vi "array -- smart enum.vi"(6 "Array of keys":string[](array[string]), 7 "hash action":T1, 9 "index IN":i32, 10 "hash key":string, 11 "hash":refnum<vi>) -> (0 "found?":bool, 1 "index OUT":i32, 2 "hash key OUT":string, 3 "hash OUT":refnum<vi>, 4 "Array of keys OUT":string[](array[string]))   [LabVIEW 2012]
uses:
  hash action control.ctl
  stack action -- control.ctl
panel:
  in  "angle":u16(ring) items=["-54", "-49.5", "-45", "-40.5", "-36", "-27", "-18", "-9", "0", "9", "18", "27", "36", "40.5", "45", "49.5", "54", "58.5", "63"]
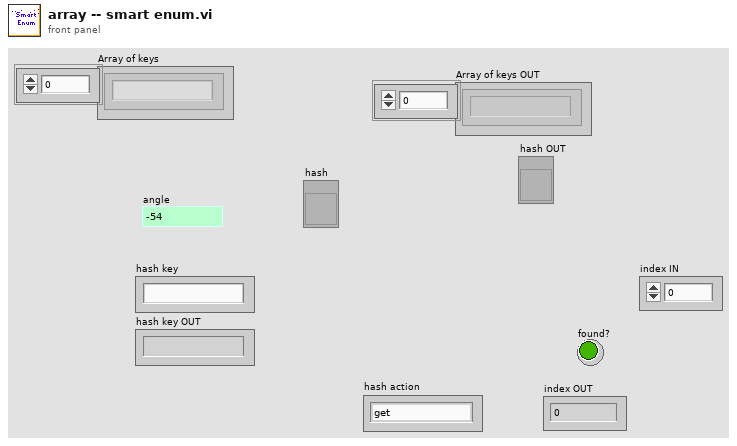
[diagram p1: front panel]
types:
  T1 = typedef "hash action control.ctl" = enum16{"get", "new", "--void", "delete", "delete all", "set", "--delete if exists", "--create if not there", "list keys", "index forw", "index back", "check", "index set", "find key"}
  T2 = typedef "stack action -- control.ctl" = enum16{"push", "pop", "check", "init"}
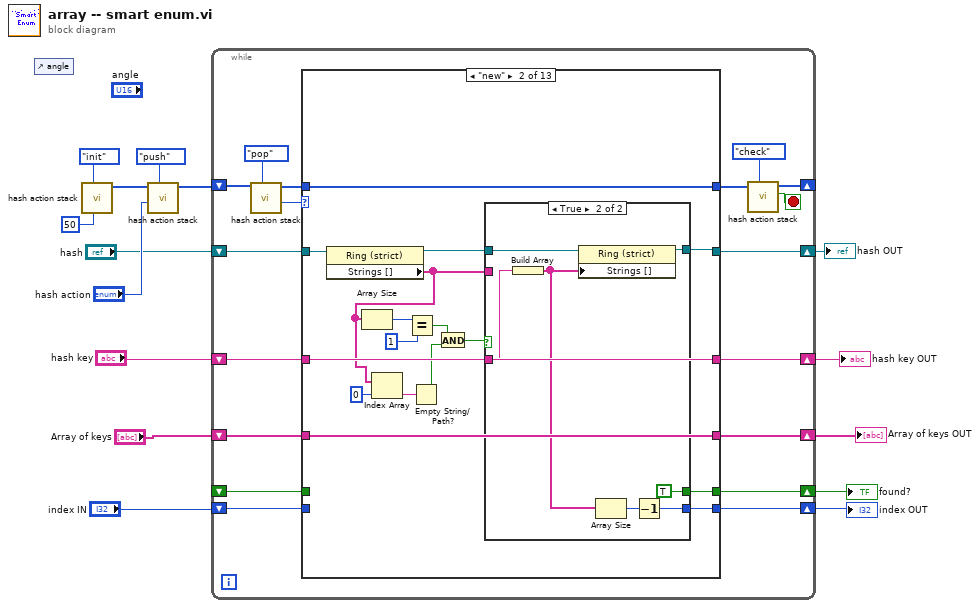
[diagram p0: block diagram]
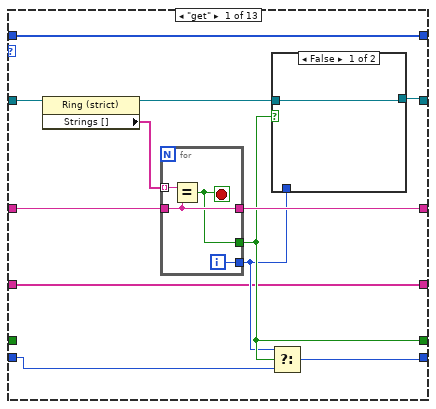
[diagram p2: hidden frame]
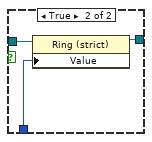
[diagram p3: hidden frame]
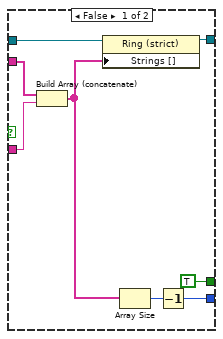
[diagram p4: hidden frame]
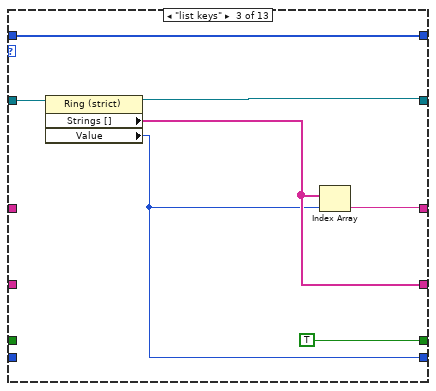
[diagram p5: hidden frame]
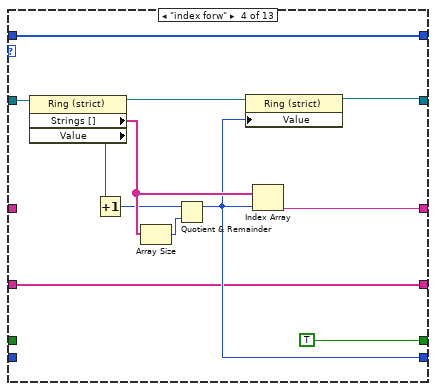
[diagram p6: hidden frame]
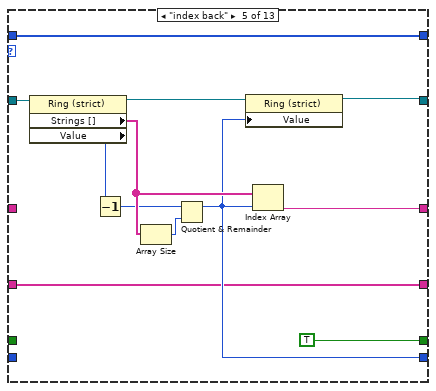
[diagram p7: hidden frame]
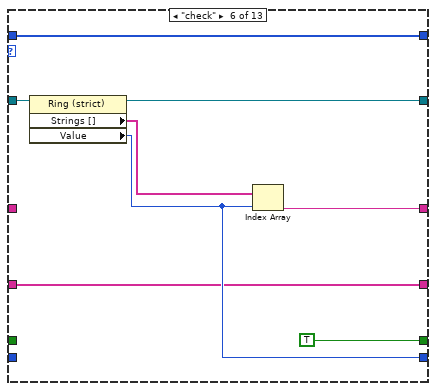
[diagram p8: hidden frame]
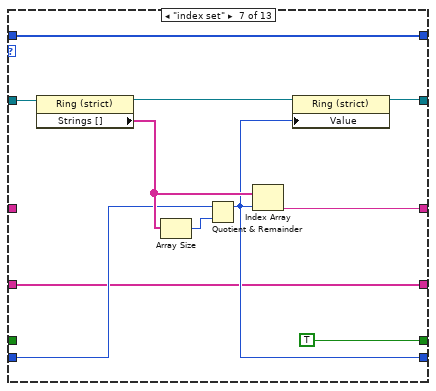
[diagram p9: hidden frame]
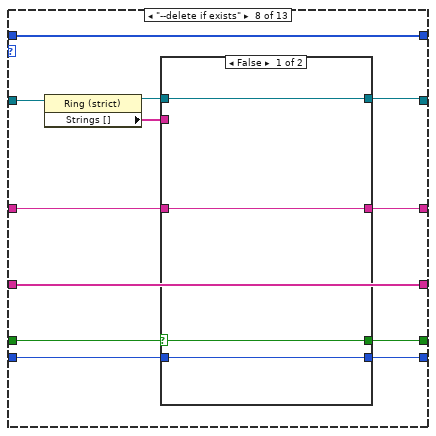
[diagram p10: hidden frame]
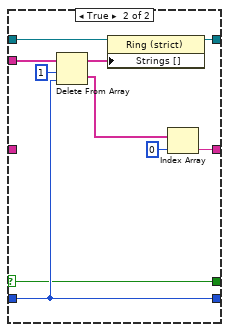
[diagram p11: hidden frame]
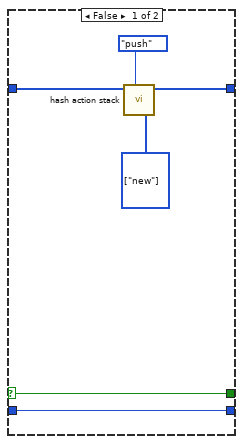
[diagram p13: hidden frame]
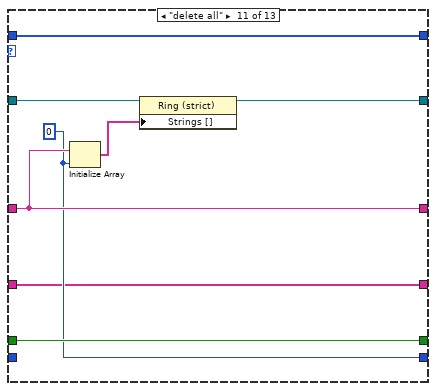
[diagram p15: hidden frame]
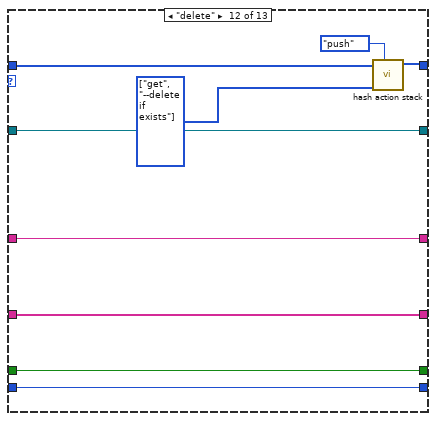
[diagram p16: hidden frame]
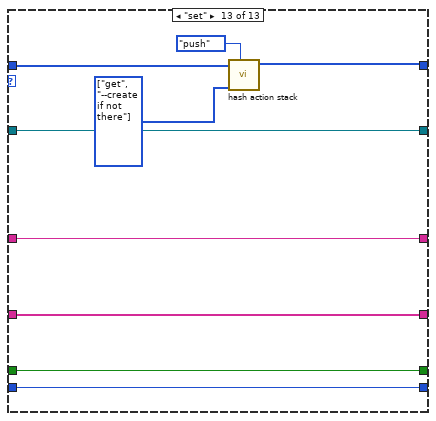
[diagram p17: hidden frame]
diagram:
  n1 = control-ref of="angle"() -> ()  [unwired: 1 out]
  n2 = call "hash action stack.vi"("init size"=50 ("dimension size"), "stack action"=stack_action_--_control."init") -> ("command stack out"=w11:T1[])  [unwired: 7 in, 2 out]
  n3 = call "hash action stack.vi"("stack action"=stack_action_--_control."push", "hash action"="hash action", "command stack"=w11) -> ("command stack out"=w13:T1[])  [unwired: 6 in, 2 out]
  n4 = while {
    shift-right: [w27] -> _
    shift-left: w13 -> [w26]
    shift-right: [w24] -> w8
    shift-left: "index IN" -> [w19]
    shift-right: [w25] -> w9
    shift-left: _ -> [w20]
    shift-right: [w18] -> w3
    shift-left: "hash" -> [w21]
    shift-right: [w23] -> w6
    shift-left: "hash key" -> [w22]
    shift-right: [w17] -> w2
    shift-left: "Array of keys" -> [w16]
    stop <- w28 stop-if-true
    n5 = call "hash action stack.vi"("stack action"=stack_action_--_control."pop", "command stack"=w26) -> ("cursor window action out"=w29:T1, "command stack out"=w32:T1[])  [unwired: 7 in, 1 out]
    n6 = case shown="\"new\"" w29 {
      tunnel: w32 -> [w45 w69 w91 w103 w115 w123 w134 w146 w164 w184 w192 w196 w205]
      tunnel: [w45 w69 w91 w103 w115 w123 w134 w146 w163 w184 w192 w195 w204] -> w30
      tunnel: w21 -> [w42 w67 w89 w101 w113 w121 w132 w139 w162 w180 w190 w194 w203]
      tunnel: w22 -> [w44 w64 _ _ _ _ _ w140 w169 w183 w189 w201 w210]
      tunnel: [w38 w68 TRUE TRUE TRUE TRUE TRUE w142 w165 w182 w191 w200 w209] -> w25
      tunnel: [w40 w63 w86 w93 w105 w118 w125 w143 w166 w181 w186 w199 w208] -> w24
      tunnel: [w43 w64 w85 w97 w109 w120 w131 w141 w169 w183 w189 w201 w210] -> w23
      tunnel: w20 -> [_ _ _ _ _ _ _ w144 w167 w182 w191 w200 w209]
      tunnel: w19 -> [w39 _ _ _ _ _ w128 w145 w168 w181 _ w199 w208]
      tunnel: [w36 w65 w88 w99 w111 w117 w126 w136 w162 w180 w187 w194 w203] -> w18
      tunnel: [w34 w62 w87 w92 w104 w116 w124 w135 w161 w179 w185 w193 w202] -> w17
      tunnel: w16 -> [w34 w62 _ w92 w104 w116 w124 w135 w161 w179 w185 w193 w202]
      frame "get" {
        n7 = property class="Ring (strict)"(reference=w42) -> (reference out=w37:refnum<vi>, "Strings []"=w41:string[])  [unwired: 1 in, 1 out]
        n8 = for {
          tunnel: w44 -> [w52]
          tunnel: [w52] -> w43
          tunnel: w41 -> [w50] mode=indexing
          tunnel: [w53] -> w35
          tunnel: [w51] -> w38
          i -> [w53]
          stop <- w51 stop-if-true
          n9 = Equal?(x=w50, y=w52) -> (x = y?=w51:bool)
        }
        n10 = case shown="False" w38 {
          tunnel: w37 -> [w46 w49]
          tunnel: [w46 w48] -> w36
          tunnel: w35 -> [_ w47]
          frame False {
          }
          frame True {
            n11 = property class="Ring (strict)"(reference=w49, "Value"=w47) -> (reference out=w48:refnum<vi>)  [unwired: 1 in, 1 out]
          }
        }
        n12 = Select(t=w35, s=w38, f=w39) -> (s? t:f=w40:i32)
      }
      frame "new" {
        n13 = property class="Ring (strict)"(reference=w67) -> (reference out=w66:refnum<vi>, "Strings []"=w59:string[])  [unwired: 1 in, 1 out]
        n14 = Array Size(array=w59) -> (size(s)=w61:i32)
        n15 = Index Array(array=w59, index=0) -> (element=w57:string)
        n16 = Equal?(x=w61, y=1) -> (x = y?=w56:bool)
        n17 = Empty String/Path?(string/path=w57) -> (empty?=w55:bool)
        n18 = And(x=w56, y=w55) -> (x .and. y?=w54:bool)
        n19 = case shown="True" w54 {
          tunnel: [TRUE TRUE] -> w68
          tunnel: w66 -> [w75 w82]
          tunnel: [w74 w81] -> w65
          tunnel: w64 -> [w73 w80]
          tunnel: w59 -> [w72 _]
          tunnel: [w71 w79] -> w63
          frame False {
            n20 = Build Array (concatenate)(w72, w73) -> (w70:string[])
            n21 = property class="Ring (strict)"(reference=w75, "Strings []"=w70) -> (reference out=w74:refnum<vi>)  [unwired: 1 in, 1 out]
            n22 = Array Size(array=w70) -> (size(s)=w77:i32)
            n23 = Decrement(x=w77) -> (x-1=w71:i32)
          }
          frame True {
            n24 = Build Array(w80) -> (w78:string[])
            n25 = property class="Ring (strict)"(reference=w82, "Strings []"=w78) -> (reference out=w81:refnum<vi>)  [unwired: 1 in, 1 out]
            n26 = Array Size(array=w78) -> (size(s)=w84:i32)
            n27 = Decrement(x=w84) -> (x-1=w79:i32)
          }
        }
      }
      frame "list keys" {
        n28 = property class="Ring (strict)"(reference=w89) -> (reference out=w88:refnum<vi>, "Strings []"=w87:string[], "Value"=w86:u16)  [unwired: 1 in, 1 out]
        n29 = Index Array(array=w87, index=w86) -> (element=w85:string)
      }
      frame "index forw" {
        n30 = property class="Ring (strict)"(reference=w101) -> (reference out=w100:refnum<vi>, "Strings []"=w96:string[], "Value"=w98:u16)  [unwired: 1 in, 1 out]
        n31 = Increment(x=w98) -> (x+1=w95:u16)
        n32 = Array Size(array=w96) -> (size(s)=w94:i32)
        n33 = Quotient & Remainder(x=w95, y=w94) -> (x-y*floor(x/y)=w93:i32)  [unwired: 1 out]
        n34 = property class="Ring (strict)"(reference=w100, "Value"=w93) -> (reference out=w99:refnum<vi>)  [unwired: 1 in, 1 out]
        n35 = Index Array(array=w96, index=w93) -> (element=w97:string)
      }
      frame "index back" {
        n36 = property class="Ring (strict)"(reference=w113) -> (reference out=w112:refnum<vi>, "Strings []"=w108:string[], "Value"=w110:u16)  [unwired: 1 in, 1 out]
        n37 = Decrement(x=w110) -> (x-1=w107:u16)
        n38 = Array Size(array=w108) -> (size(s)=w106:i32)
        n39 = Quotient & Remainder(x=w107, y=w106) -> (x-y*floor(x/y)=w105:i32)  [unwired: 1 out]
        n40 = property class="Ring (strict)"(reference=w112, "Value"=w105) -> (reference out=w111:refnum<vi>)  [unwired: 1 in, 1 out]
        n41 = Index Array(array=w108, index=w105) -> (element=w109:string)
      }
      frame "check" {
        n42 = property class="Ring (strict)"(reference=w121) -> (reference out=w117:refnum<vi>, "Strings []"=w119:string[], "Value"=w118:u16)  [unwired: 1 in, 1 out]
        n43 = Index Array(array=w119, index=w118) -> (element=w120:string)
      }
      frame "index set" {
        n44 = property class="Ring (strict)"(reference=w132) -> (reference out=w127:refnum<vi>, "Strings []"=w130:string[])  [unwired: 1 in, 1 out]
        n45 = Array Size(array=w130) -> (size(s)=w129:i32)
        n46 = Quotient & Remainder(x=w128, y=w129) -> (x-y*floor(x/y)=w125:i32)  [unwired: 1 out]
        n47 = Index Array(array=w130, index=w125) -> (element=w131:string)
        n48 = property class="Ring (strict)"(reference=w127, "Value"=w125) -> (reference out=w126:refnum<vi>)  [unwired: 1 in, 1 out]
      }
      frame "--delete if exists" {
        n49 = property class="Ring (strict)"(reference=w139) -> (reference out=w137:refnum<vi>, "Strings []"=w138:string[])  [unwired: 1 in, 1 out]
        n50 = case shown="False" w144 {
          selector: w144 -> [w150 w158]
          tunnel: w145 -> [w149 w159]
          tunnel: [w149 w159] -> w143
          tunnel: [w150 w158] -> w142
          tunnel: [w148 w151] -> w141
          tunnel: w140 -> [w148 _]
          tunnel: w138 -> [_ w156]
          tunnel: w137 -> [w147 w155]
          tunnel: [w147 w154] -> w136
          frame False {
          }
          frame True {
            n51 = Delete From Array(array=w156, length=1, index=w159) -> (deleted portion=w152:string[], array with subset deleted=w153:string[])
            n52 = property class="Ring (strict)"(reference=w155, "Strings []"=w153) -> (reference out=w154:refnum<vi>)  [unwired: 1 in, 1 out]
            n53 = Index Array(array=w152, index=0) -> (element=w151:string)
          }
        }
      }
      frame "--create if not there" {
        n54 = case shown="True" w167 {
          selector: w167 -> [w174 w178]
          tunnel: w168 -> [w175 w176]
          tunnel: [w175 w176] -> w166
          tunnel: [w174 w178] -> w165
          tunnel: w164 -> [w172 w177]
          tunnel: [w171 w177] -> w163
          frame False {
            w170 = T1[] [enum."new"] items=["get", "new", "--void", "delete", "delete all", "set", "--delete if exists", "--create if not there", "list keys", "index forw", "index back", "check", "index set", "find key"] ("hash action list")
            n55 = call "hash action stack.vi"("stack action"=stack_action_--_control."push", "hash action list"=w170, "command stack"=w172) -> ("command stack out"=w171:T1[])  [unwired: 6 in, 2 out]
          }
          frame True {
          }
        }
      }
      frame "--void", Default {
      }
      frame "delete all" {
        w186 = 0
        n56 = Initialize Array(w189, w186) -> (w188:string[])
        n57 = property class="Ring (strict)"(reference=w190, "Strings []"=w188) -> (reference out=w187:refnum<vi>)  [unwired: 1 in, 1 out]
      }
      frame "delete" {
        w197 = T1[] [enum."get", enum."--delete if exists"] items=["get", "new", "--void", "delete", "delete all", "set", "--delete if exists", "--create if not there", "list keys", "index forw", "index back", "check", "index set", "find key"] ("hash action list")
        n58 = call "hash action stack.vi"("stack action"=stack_action_--_control."push", "hash action list"=w197, "command stack"=w196) -> ("command stack out"=w195:T1[])  [unwired: 6 in, 2 out]
      }
      frame "set" {
        w206 = T1[] [enum."get", enum."--create if not there"] items=["get", "new", "--void", "delete", "delete all", "set", "--delete if exists", "--create if not there", "list keys", "index forw", "index back", "check", "index set", "find key"] ("hash action list")
        n59 = call "hash action stack.vi"("stack action"=stack_action_--_control."push", "hash action list"=w206, "command stack"=w205) -> ("command stack out"=w204:T1[])  [unwired: 6 in, 2 out]
      }
    }
    n60 = call "hash action stack.vi"("stack action"=stack_action_--_control."check", "command stack"=w30) -> ("stack is empty ?"=w28:bool, "command stack out"=w27:T1[])  [unwired: 7 in, 1 out]
  }
  "found?" <- w9
  "index OUT" <- w8
  "hash key OUT" <- w6
  "hash OUT" <- w3
  "Array of keys OUT" <- w2
